vi "Open Local.vi"(8 "error in (no error)":errorcluster) -> (0 "error out":errorcluster, 2 "Device Name":string, 3 "LINX Client out":refnum<class "LINX Client.lvclass">)   [LabVIEW 2020, in "LINX Client.lvclass"]
uses:
  LINX Client.lvclass
  LINX Base.lvclass
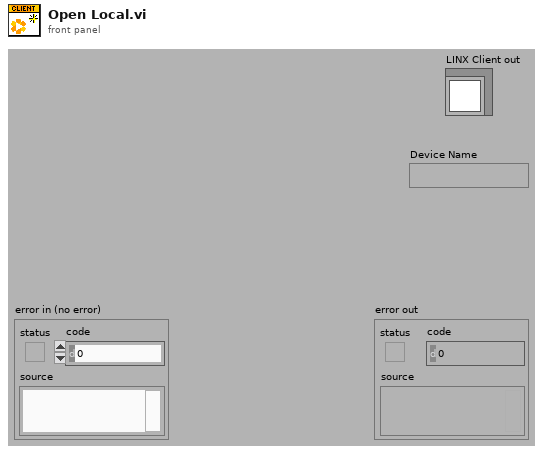
[diagram p1: front panel]
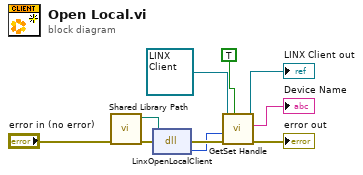
[diagram p0: block diagram]
diagram:
  n1 = call "Shared Library Path.vi"("error in (no error)"="error in (no error)") -> ("error out"=w9:errorcluster, "Path"=w8:path)  [unwired: 9 out]
  n2 = dll-call lib="Z:/Development/LabVIEW Hobbyist Toolkit/LabVIEW/vi.lib/MakerHub/LINX/Resources/libLinxDevice.dll" fn="LinxOpenLocalClient"(path in=w8, error in=w9) -> (error out=w7:errorcluster, "LinxDevice"=w3:u64)  [unwired: 1 in, 1 out]
  n3 = call-dynamic "GetSet Handle.vi"("store (F)"=TRUE, "error in"=w7, "handle in"=w3, "LINX Base in"=refnum<class "LINX Client.lvclass"> refnum ("LINX Device")) -> ("error out"=→"error out":errorcluster, "name"=→"Device Name":string, "LINX Base out"=→"LINX Client out":refnum<class "LINX Client.lvclass">)  [unwired: 1 in, 4 out]
